vi "LensMotors_go_to_position.vi"(7 "modIdTag":string="S1", 8 "error in (no error)":errorcluster, 10 "position":sgl, 11 "channel":refnum<k24>) -> (0 "error out":errorcluster)   [LabVIEW 2021]
uses:
  F:/2PhotonVision/psychometric_function_v2/lib/Grpc.Core.dll
  lib/Grpc.Core.dll
  F:/2PhotonVision/psychometric_function_v2/lib/FossilProtosSharp.dll
  lib/FossilProtosSharp.dll
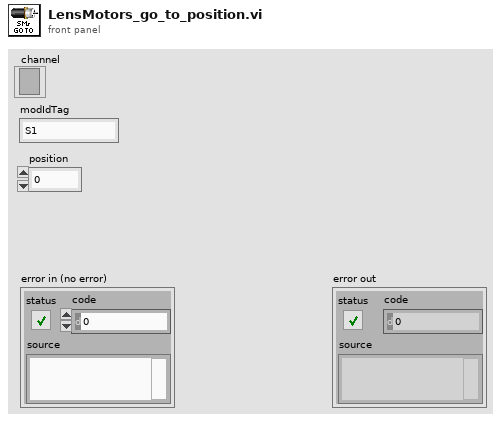
[diagram p1: front panel]
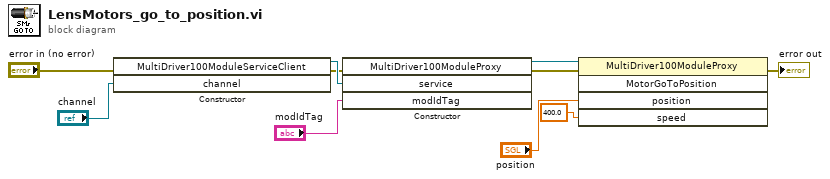
[diagram p0: block diagram]
diagram:
  n1 = constructor class="MultiDriver100ModuleServiceClie"(error in="error in (no error)", "channel"="channel") -> (reference out=w8:refnum<k24>, error out=w7:errorcluster)  [unwired: 2 in, 2 out]
  n2 = constructor class="MultiDriver100ModuleProxy"(error in=w7, "service"=w8, "modIdTag"="modIdTag") -> (reference out=w1:refnum<k24>, error out=w2:errorcluster)  [unwired: 2 in, 3 out]
  n3 = invoke class="MultiDriver100ModuleProxy" method="MotorGoToPosition"(reference=w1, error in=w2, "position"="position", "speed"=sgl 400.0) -> (error out=→"error out":errorcluster)  [unwired: 1 in, 4 out]
